vi "new mag tester.vi"() -> ()   [LabVIEW 2017]
uses:
  typedefs/commandType.ctl
  typedefs/transmit code.ctl
panel:
  out "MAG 5":cluster{"x":sgl, "y":sgl, "z":sgl}(graph)
  out "MAG 4":cluster{"x":sgl, "y":sgl, "z":sgl}(graph)
  out "MAG 3":cluster{"x":sgl, "y":sgl, "z":sgl}(graph)
  out "MAG 2":cluster{"x":sgl, "y":sgl, "z":sgl}(graph)
  out "MAG 1":cluster{"x":sgl, "y":sgl, "z":sgl}(graph)
  out "MAG 0":cluster{"x":sgl, "y":sgl, "z":sgl}(graph)
  out "stop2":bool
  in  "stop":bool
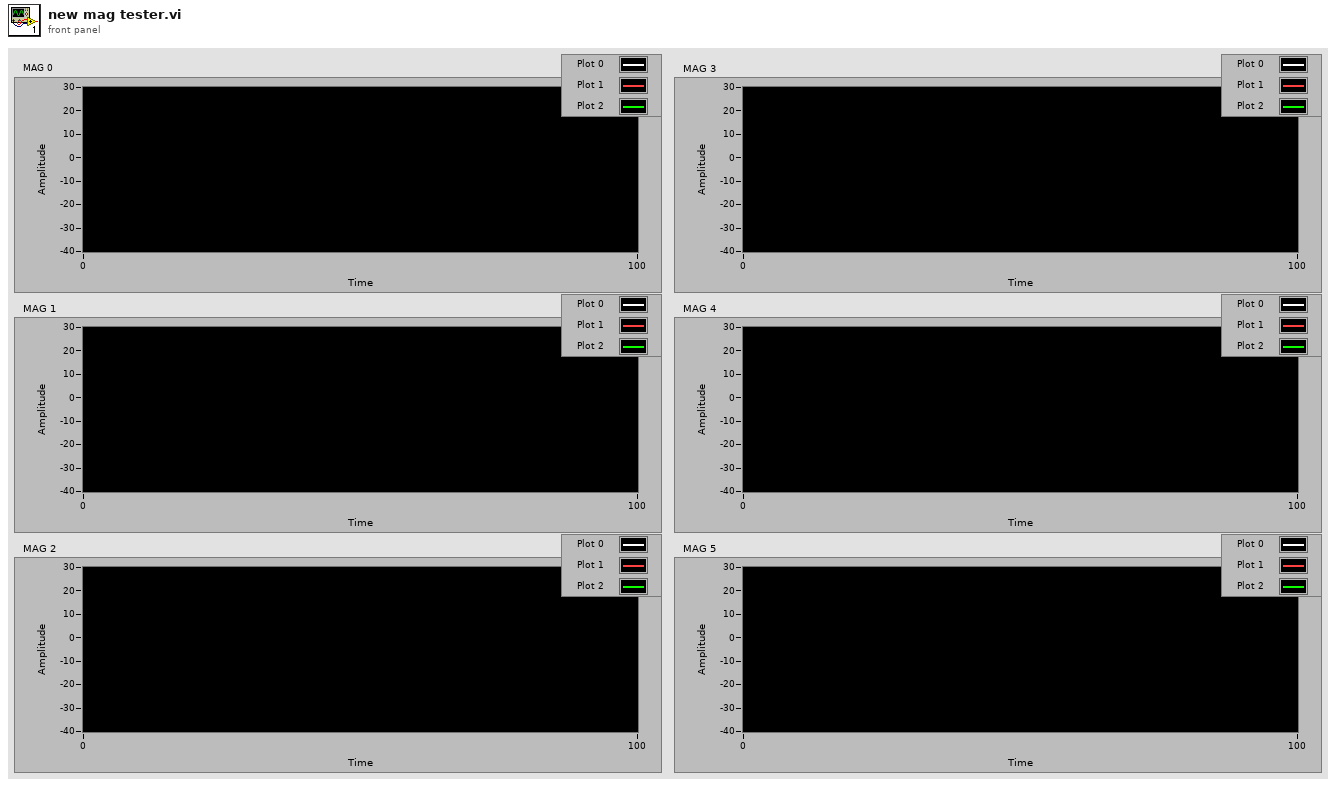
[diagram p1: front panel]
types:
  T1 = typedef "commandType.ctl" = enum16{"G - set gain", "C - activate coil", "D - deactivate coil", "L - set LED", "A - set AUTO", "V - set verbose", "T - set transmission", "R - get version", "Z - zero accelerometer", "F - set auto-flash led", "X - synchronize serial", "Q - reset queues and timers", "S - save configuration"}
  T2 = typedef "transmit code.ctl" = u16
  T3 = typedef "queue cluster.ctl" = cluster{"voltage":T4, "coil":T4, "mag":T4, "accel":T4, "crossing":T4, "angle":T4, "pulse":T4}
  T4 = typedef "reading queue.ctl" = refnum<queue>
  T5 = typedef "reading.ctl" = cluster{"reading type":T6, "time":fxp<+,48,48>, "x":sgl, "y":sgl, "z":sgl, "XSUM":u8}
  T6 = typedef "readingType.ctl" = enum8{"SYNC", "DETVAL", "COILI", "MAGVEC", "ACCVEC", "CROSSING"}
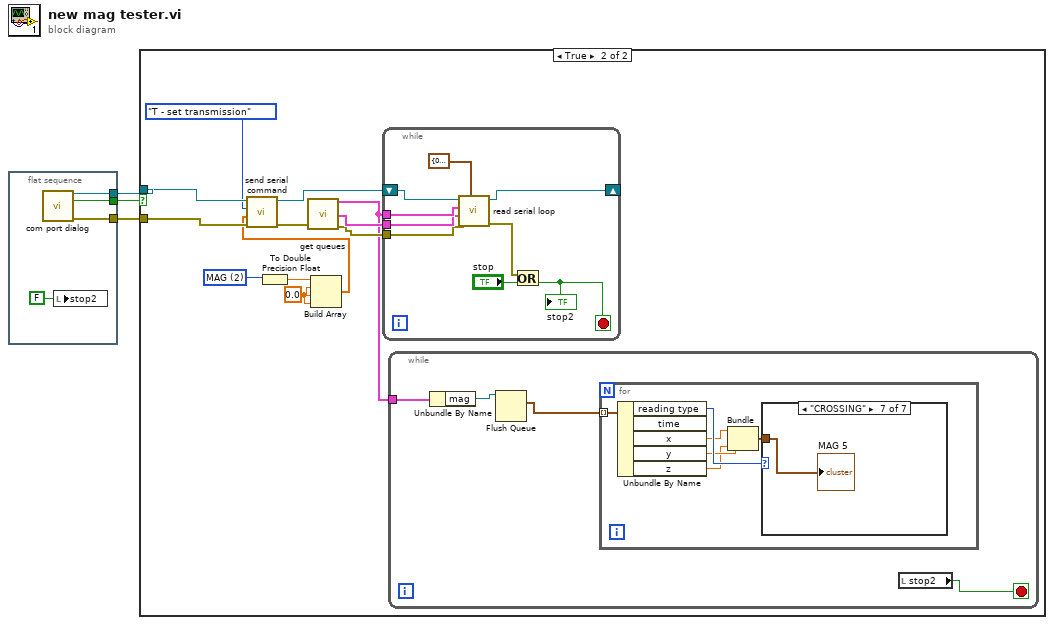
[diagram p0: block diagram]
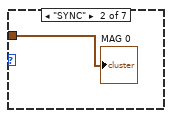
[diagram p4: hidden frame]
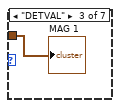
[diagram p5: hidden frame]
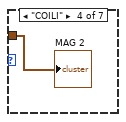
[diagram p6: hidden frame]
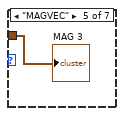
[diagram p7: hidden frame]
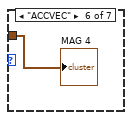
[diagram p8: hidden frame]
diagram:
  n1 = flat-sequence {
    tunnel: [w7] -> w3
    tunnel: [w6] -> w2
    tunnel: [w5] -> w1
    frame #0 {
      n2 = call "com port dialog.vi"() -> ("VISA resource name out"=w5:refnum<visa-resource-name>, "port opened"=w7:bool, "error out"=w6:errorcluster)  [unwired: 11 in, 2 out]
      n3 = local write "stop2"(FALSE ("stop2")) -> ()
    }
  }
  n4 = case shown="True" w3 {
    tunnel: w2 -> [_ w19]
    tunnel: w1 -> [_ w18]
    frame False {
    }
    frame True {
      w13 = 0.0 ("element")
      w16 = T2 2 items=["ADC"=1, "MAG"=2, "ACC"=4, "COIL"=8, "CROSSING"=16] ("Ring")
      n5 = To Double Precision Float(number=w16) -> (double precision float=w15:dbl)
      n6 = Build Array(w15, w13, w13, w13) -> (w14:dbl[])
      n7 = call "send serial command.vi"("error in (no error)"=w19, "data"=w14, "Command"=commandType."T - set transmission", "visa resource"=w18) -> ("error out"=w12:errorcluster, "VISA resource name out"=w9:refnum<visa-resource-name>)  [unwired: 5 in, 1 out]
      n8 = call "get queues.vi"("error in (no error)"=w12) -> ("display queues"=w8:T3, "disk queues"=w11:T3, "error out"=w10:errorcluster)  [unwired: 12 in]
      n9 = while {
        tunnel: w8 -> [w44]
        tunnel: w11 -> [w43]
        tunnel: w10 -> [w42]
        shift-right: [w41] -> _
        shift-left: w9 -> [w40]
        stop <- w38 stop-if-true
        n10 = call "read serial loop.vi"("earth magnetic field"=cluster{"x":sgl, "y":sgl, "z":sgl} {"x"=0.0, "y"=0.0, "z"=0.0}, "error in (no error)"=w42, "disk queues"=w43, "display queues"=w44, "serial port"=w40) -> ("error out"=w37:errorcluster, "VISA resource name out"=w41:refnum<visa-resource-name>)  [unwired: 3 in, 2 out]
        n11 = Or(x=w37, y="stop") -> (x .or. y?=w38:bool)
        "stop2" <- w38
      }
      n12 = while {
        tunnel: w8 -> [w23]
        stop <- w20 stop-if-true
        n13 = Unbundle By Name(w23) -> ("mag"=w22:T4)
        n14 = Flush Queue(queue=w22) -> (remaining elements=w21:T5[])  [unwired: 1 in, 2 out]
        n15 = for {
          tunnel: w21 -> [w29] mode=indexing
          n16 = Unbundle By Name(w29) -> ("reading type"=w28:T6, "x"=w27:sgl, "y"=w26:sgl, "z"=w25:sgl)  [unwired: 1 out]
          n17 = Bundle("x"=w27, "y"=w26, "z"=w25) -> (w24:cluster{"x":sgl, "y":sgl, "z":sgl})  [unwired: 1 in]
          n18 = case shown="\"MAGVEC5\"" w28 {
            tunnel: w24 -> [_ w30 w31 w32 w33 w34 w35]
            frame "SYNC", Default {
            }
            frame "SYNC" {
              "MAG 0" <- w30
            }
            frame "DETVAL" {
              "MAG 1" <- w31
            }
            frame "COILI" {
              "MAG 2" <- w32
            }
            frame "MAGVEC" {
              "MAG 3" <- w33
            }
            frame "ACCVEC" {
              "MAG 4" <- w34
            }
            frame "CROSSING" {
              "MAG 5" <- w35
            }
          }
        }
        n19 = local read "stop2"() -> (w20:bool)
      }
    }
  }
